vi "ExportSPadToTest.vi"(11 "Settings":T1={"Name of test"="", "Date"=timestamp(0 s since 1904-01-01), "Location"="", "Template"="", "Soundcard"="", "resolution"=32, "Sampling rate"=48000, "Ch1 Gain "=25.0, "Ch2 Gain"=10.0, "Sample time (s)"=0.3, "Pre-trigger (s)"=0.01, "Hammer Threshold"=10.0, "Positions"=12, "Taps/Position"=5, "Set Names"="", "Freq resolution"=10.0, "Hammer cutoff"=0.0, "Mic cutoff"=0.0, "Double bounce "=0.0, "Hammer Cal"=10.0, "dB Offset"=0.0, "Accel Cal"=10.0, "Vibrometer Cal"=0.0, "Mic Cal"=0.0, "Output"=2, "Voltage Cal"=1.0, "Vibrometer Port"="ASRL27::INSTR", "Range"=4, "High Pass"=2, "Bandwidth"=4, "X Range"=[], "Y Range"=[], "dB Spread"=0.0, "Trigger"=0, "Ch_1"=25, "Ch_2"=25, "flip?"=FALSE, "60Hz"=FALSE, "Time offset"=0.0, "Piezo Cal"=1.0, "Default Notes"=""} {"Ch_2" min=1 step=1; "Ch_1" min=1 max=100 step=1; "Trigger" items=["Hammer (force)", "Self-tap", "Spacebar"]; "Bandwidth" items=["1 kHz"=1, "5 kHz"=5, "10 kHz"=10, "25 kHz"=25, "50 kHz"=50, "100 kHz"=100]; "High Pass" items=["Off", "13 Hz", "104 Hz"]; "Range" items=["10 mm/s"=1, "20 mm/s"=2, "50 mm/s"=5, "100 mm/s"=10, "200 mm/s"=20, "500 mm/s"=50, "1 m/s"=100, "2 m/s"=200]; "Output" items=["Accelerometer", "Speed (from acceleration)", "Microphone", "Vibrometer", "Piezo"]; "Voltage Cal" format="%#_13g"; "Ch2 Gain" format="%#_13g"; "Ch1 Gain" format="%#_13g"; "Double bounce" min=0.0; "Mic cutoff" min=0.0 format="%#_4g"; "Hammer cutoff" min=0.0 format="%#_4g"; "Freq resolution" min=0.0; "Pre-trigger (s)" format="%#_13g"; "Date" format="%<%H:%M\n%d/%m/%y>T"; "resolution" items=["16 bit"=16, "24 bit"=24, "32 bit"=32]; "Sampling rate" items=["22050 samp/s"=22050, "44100 samp/s"=44100, "48000 samp/s"=48000]}) -> (2 "Success":bool, 3 "Settings Out":T1={"Name of test"="", "Date"=timestamp(0 s since 1904-01-01), "Location"="", "Template"="", "Soundcard"="", "resolution"=32, "Sampling rate"=48000, "Ch1 Gain "=25.0, "Ch2 Gain"=10.0, "Sample time (s)"=0.3, "Pre-trigger (s)"=0.01, "Hammer Threshold"=10.0, "Positions"=12, "Taps/Position"=5, "Set Names"="", "Freq resolution"=10.0, "Hammer cutoff"=0.0, "Mic cutoff"=0.0, "Double bounce "=0.0, "Hammer Cal"=1.0, "dB Offset"=0.0, "Accel Cal"=1.0, "Vibrometer Cal"=1.0, "Mic Cal"=1.0, "Output"=2, "Voltage Cal"=1.0, "Vibrometer Port"="ASRL27::INSTR", "Range"=4, "High Pass"=2, "Bandwidth"=4, "X Range"=[], "Y Range"=[], "dB Spread"=0.0, "Trigger"=0, "Ch_1"=1, "Ch_2"=2, "flip?"=FALSE, "60Hz"=FALSE, "Time offset"=0.0, "Piezo Cal"=1.0, "Default Notes"=""} {"Ch_2" min=1 step=1; "Ch_1" min=1 max=100 step=1; "Trigger" items=["Hammer (force)", "Self-tap", "Spacebar"]; "Bandwidth" items=["1 kHz"=1, "5 kHz"=5, "10 kHz"=10, "25 kHz"=25, "50 kHz"=50, "100 kHz"=100]; "High Pass" items=["Off", "13 Hz", "104 Hz"]; "Range" items=["10 mm/s"=1, "20 mm/s"=2, "50 mm/s"=5, "100 mm/s"=10, "200 mm/s"=20, "500 mm/s"=50, "1 m/s"=100, "2 m/s"=200]; "Output" items=["Accelerometer", "Speed (from acceleration)", "Microphone", "Vibrometer", "Piezo"]; "Voltage Cal" format="%#_13g"; "Ch2 Gain" format="%#_13g"; "Ch1 Gain" format="%#_13g"; "Double bounce" min=0.0; "Mic cutoff" min=0.0 format="%#_4g"; "Hammer cutoff" min=0.0 format="%#_4g"; "Freq resolution" min=0.0; "Pre-trigger (s)" format="%#_13g"; "Date" format="%<%H:%M\n%d/%m/%y>T"; "resolution" items=["16 bit"=16, "24 bit"=24, "32 bit"=32]; "Sampling rate" items=["22050 samp/s"=22050, "44100 samp/s"=44100, "48000 samp/s"=48000]})   [LabVIEW 2022 SP3]
uses:
  PreferencesControl.ctl
  <vilib>/Utility/miscctls.llb/LVSelectionTypeDef.ctl
  <vilib>/Utility/error.llb/Trim Whitespace One-Sided.vi
panel:
  in  "Instrument Notes":string
  in  "Instrument Name":string(combo)
  in  "Test Name":string
  out "File name":string
  in  "Tag List":bool
  in  "Instrument Keywords":string
  in  "OK Button":bool
  in  "Cancel Button":bool
  # "Export to New Test"
  # "Hz"
  # "dB"
  # "dB"
  # "sec"
  # "sec"
  # "mV/Pa"
  # "mV/m/s2"
  # "mV/mm/s"
  # "V/N"
  # "sec"
  # "sec"
  # "mV/N"
  # "a.u."
  # "a.u."
  # "sec"
  # "Hz"
  # "dB"
  # "dB"
  # "sec"
  # "sec"
  # "mV/Pa"
  # "mV/m/s2"
  # "mV/mm/s"
  # "V/N"
  # "sec"
  # "sec"
  # "mV/N"
  # "a.u."
  # "a.u."
  # "sec"
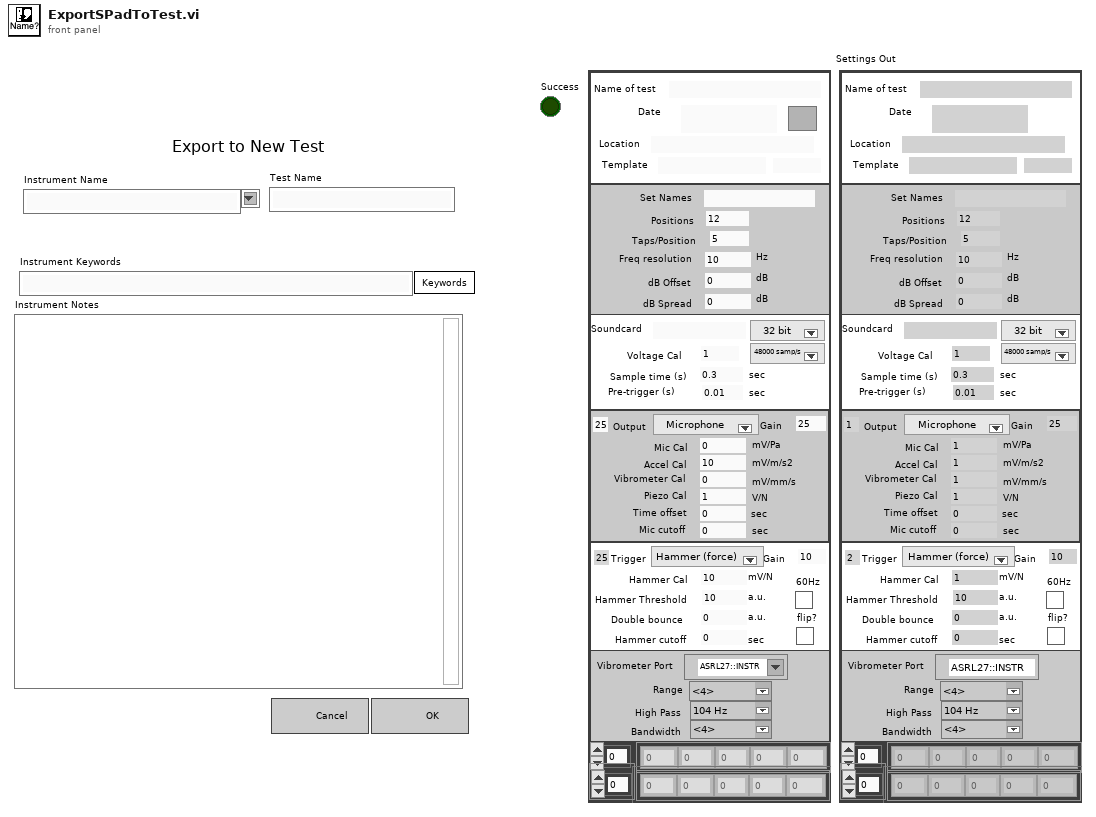
[diagram p1: front panel]
types:
  T1 = typedef "PreferencesControl.ctl" = cluster{"Name of test":string, "Date":timestamp, "Location":string, "Template":string, "Soundcard":string, "resolution":u16, "Sampling rate":u16, "Ch1 Gain ":dbl, "Ch2 Gain":dbl, "Sample time (s)":dbl, "Pre-trigger (s)":dbl, "Hammer Threshold":dbl, "Positions":i16, "Taps/Position":i16, "Set Names":string, "Freq resolution":dbl, "Hammer cutoff":dbl, "Mic cutoff":dbl, "Double bounce ":dbl, "Hammer Cal":dbl, "dB Offset":dbl, "Accel Cal":dbl, "Vibrometer Cal":dbl, "Mic Cal":dbl, "Output":u16, "Voltage Cal":dbl, "Vibrometer Port":refnum<visa-resource-name>, "Range":u16, "High Pass":u16, "Bandwidth":u16, "X Range":cluster{"Minimum":dbl, "Maximum":dbl, "Increment":dbl, "Minor Increment":dbl, "Start":dbl}[], "Y Range":cluster{"Minimum":dbl, "Maximum":dbl, "Increment":dbl, "Minor Increment":dbl, "Start":dbl}[], "dB Spread":dbl, "Trigger":u16, "Ch_1":u8, "Ch_2":u8, "flip?":bool, "60Hz":bool, "Time offset":dbl, "Piezo Cal":dbl, "Default Notes":string}
  T2 = enum8{"Enabled", "Disabled", "Disabled and Grayed Out"}
  T3 = typedef "LVSelectionTypeDef.ctl" = cluster{"Selection Start":u32, "Selection End":u32}
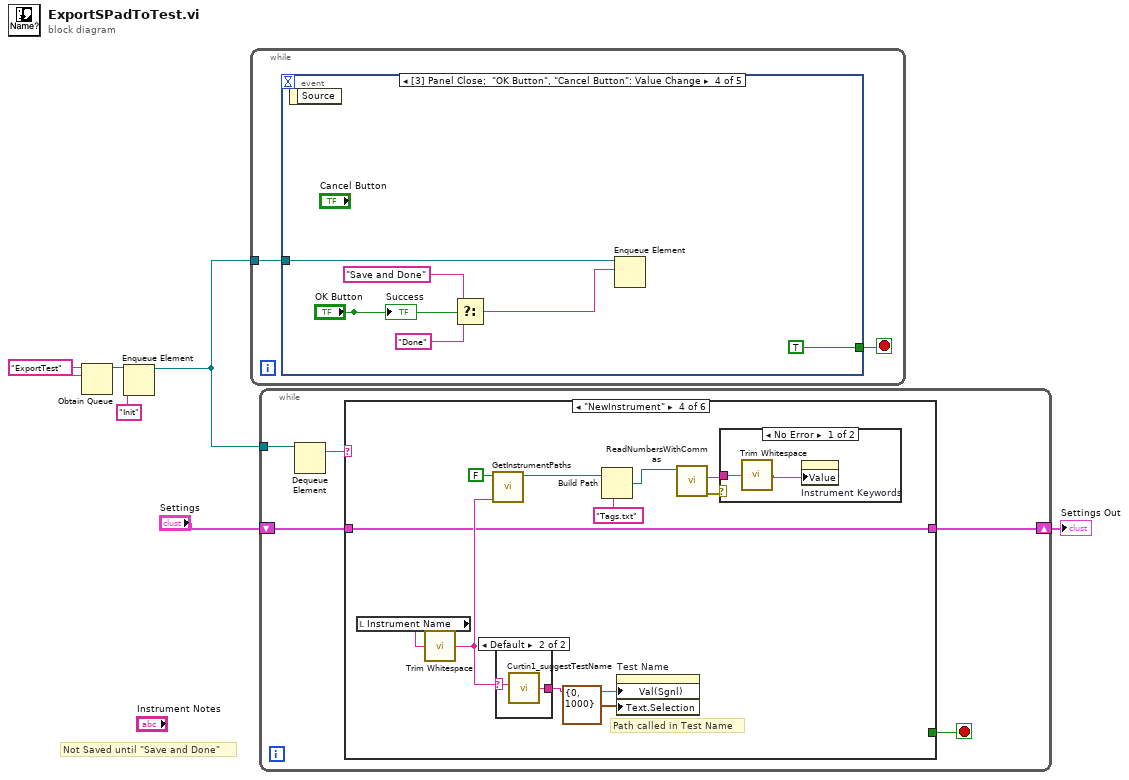
[diagram p0: block diagram]
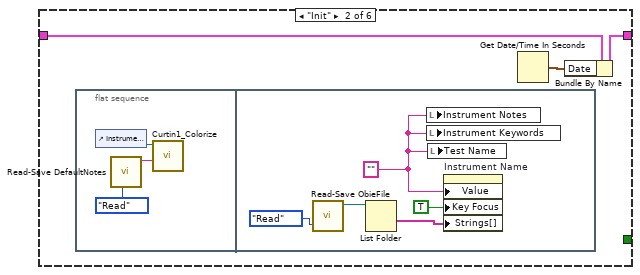
[diagram p3: hidden frame]
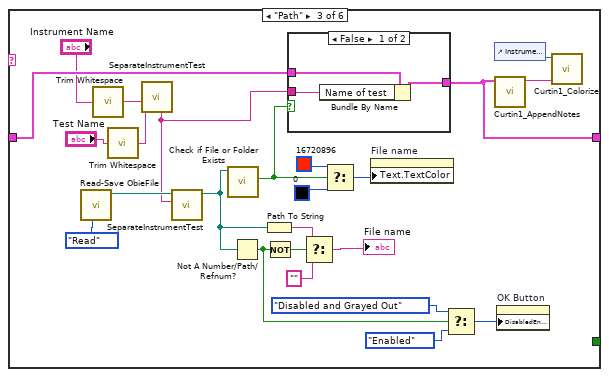
[diagram p4: hidden frame]
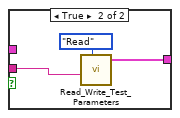
[diagram p5: hidden frame]
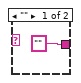
[diagram p7: hidden frame]
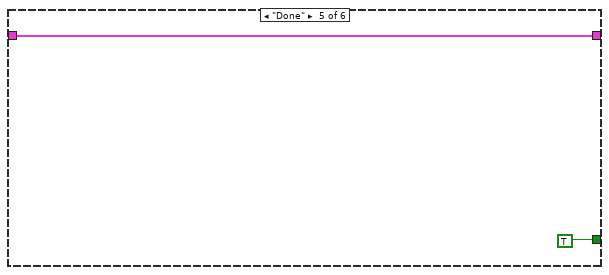
[diagram p8: hidden frame]
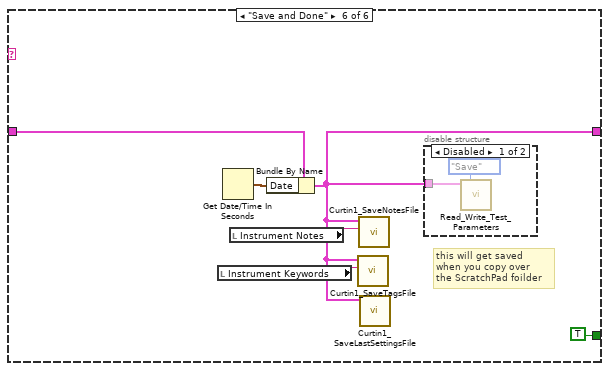
[diagram p9: hidden frame]
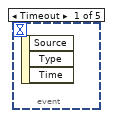
[diagram p11: hidden frame]
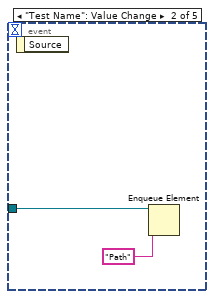
[diagram p12: hidden frame]
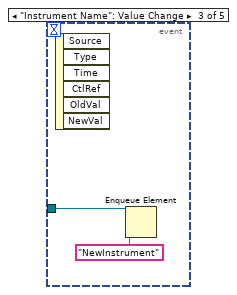
[diagram p13: hidden frame]
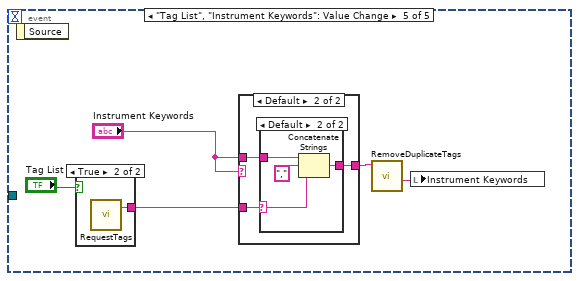
[diagram p14: hidden frame]
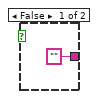
[diagram p17: hidden frame]
diagram:
  w6 = "ExportTest" ("name (unnamed)")
  # "Not Saved until \"Save and Done\""
  n1 = Obtain Queue(name (unnamed)=w6, element data type=w6) -> (queue out=w5:refnum<queue>)  [unwired: 3 in, 2 out]
  n2 = Enqueue Element(queue=w5, element="Init") -> (queue out=w3:refnum<queue>)  [unwired: 2 in, 2 out]
  n3 = while {
    tunnel: w3 -> [w7]
    stop <- w8 stop-if-true
    n4 = event shown="[3] Panel Close;  \"OK Button\", \"Cancel Button\": Value Change" {
      selector: _ -> [_ _ _ _ _]
      dyn-events: _ -> [_ _ _ _ _]
      timeout: _ -> [_ _ _ _ _]
      tunnel: [_ _ _ TRUE _] -> w8
      tunnel: w7 -> [_ w9 w11 w17 _]
      event Timeout {
        n5 = event-data() -> ()  [unwired: 1 in, 3 out]
      }
      event "Test Name": Value Change {
        n6 = event-data() -> ()  [unwired: 1 in, 1 out]
        n7 = Enqueue Element(queue=w9, element="Path") -> ()  [unwired: 2 in, 3 out]
      }
      event "Instrument Name": Value Change {
        n8 = event-data() -> ()  [unwired: 1 in, 6 out]
        n9 = Enqueue Element(queue=w11, element="NewInstrument") -> ()  [unwired: 2 in, 3 out]
      }
      event Panel Close; "OK Button", "Cancel Button": Value Change {
        n10 = event-data() -> ()  [unwired: 1 in, 1 out]
        n11 = Select(t="Save and Done" ("element"), s="OK Button", f="Done" ("element")) -> (s? t:f=w14:string)
        n12 = Enqueue Element(queue=w17, element=w14) -> ()  [unwired: 2 in, 3 out]
        "Success" <- "OK Button"
      }
      event "Tag List", "Instrument Keywords": Value Change {
        n13 = event-data() -> ()  [unwired: 1 in, 1 out]
        n14 = case shown="True" "Tag List" {
          tunnel: ["" ("Tags out") w34] -> w23
          frame False {
          }
          frame True {
            n15 = call "RequestTags.vi"() -> ("Tags out"=w34:string)  [unwired: 11 in]
          }
        }
        n16 = case shown="Default" "Instrument Keywords" {
          tunnel: w23 -> [w24 w25]
          tunnel: "Instrument Keywords" -> [_ w27]
          tunnel: [w24 w26] -> w21
          frame "" {
          }
          frame Default {
            n17 = case shown="Default" w25 {
              selector: w25 -> [_ w29]
              tunnel: w27 -> [w28 w32]
              tunnel: [w28 w31] -> w26
              frame "" {
              }
              frame Default {
                n18 = Concatenate Strings(w32, "," ("string"), w29) -> (w31:string)
              }
            }
          }
        }
        n19 = call "RemoveDuplicateTags.vi"("Tags"=w21) -> ("Tag string"=w19:string)  [unwired: 9 in, 1 out]
        n20 = local write "Instrument Keywords"(w19) -> ()
      }
    }
  }
  n21 = while {
    tunnel: w3 -> [w38]
    shift-right: [w35] -> w1
    shift-left: "Settings" -> [w36]
    stop <- w37 stop-if-true
    n22 = Dequeue Element(queue=w38) -> (element=w39:string)  [unwired: 2 in, 3 out]
    n23 = case shown="\"NewInstrument\"" w39 {
      tunnel: [_ _ _ _ TRUE TRUE] -> w37
      tunnel: w36 -> [w40 w41 w59 w85 w98 w101]
      tunnel: [w40 w43 w56 w85 w98 w100] -> w35
      frame Default {
      }
      frame "Init" {
        n24 = flat-sequence {
          frame #0 {
            n25 = control-ref of="Instrument Notes"() -> (w45:refnum<vi>)
            n26 = call "Read-Save DefaultNotes.vi"("Task"=enum16{"Save", "Read"}."Read") -> ("Notes Out"=w44:string)  [unwired: 9 in, 1 out]
            n27 = call "Curtin1_Colorize.vi"("Instrument Notes"=w44, "Text"=w45) -> ()  [unwired: 10 in]
          }
          frame #1 {
            w47 = "" ("Value (Signaling)")
            n28 = call "Read-Save ObieFile.vi"("Task"=enum16{"Save", "Read"}."Read") -> ("DataPath Out"=w50:path)  [unwired: 8 in, 2 out]
            n29 = List Folder(path=w50) -> (folder names=w51:string[])  [unwired: 3 in, 3 out]
            n30 = local write "Instrument Notes"(w47) -> ()
            n31 = local write "Instrument Keywords"(w47) -> ()
            n32 = local write "Test Name"(w47) -> ()
            n33 = property on="Instrument Name" class="CmbBox"("Value"=w47, "Key Focus"=TRUE, "Strings[]"=w51) -> ()  [unwired: 2 in, 2 out]
          }
        }
        n34 = Get Date/Time In Seconds() -> (seconds since 1Jan1904=w42:timestamp)
        n35 = Bundle By Name(cluster=w41, "Date"=w42) -> (w43:T1)
      }
      frame "Path" {
        n36 = call "Read-Save ObieFile.vi"("Task"=enum16{"Save", "Read"}."Read") -> ("DataPath Out"=w62:path)  [unwired: 8 in, 2 out]
        n37 = call <vilib>:"Trim Whitespace.vi"("string"="Instrument Name") -> ("trimmed string"=w55:string)  [unwired: 1 in]
        n38 = call <vilib>:"Trim Whitespace.vi"("string"="Test Name") -> ("trimmed string"=w52:string)  [unwired: 1 in]
        n39 = call "SeparateInstrumentTest.vi"("test in"=w52, "Instrument in"=w55) -> ("Instrument -- test out"=w60:string)  [unwired: 5 in, 4 out]
        n40 = call "SeparateInstrumentTest.vi"("Instrument"=w60, "path in"=w62) -> ("path out"=w61:path)  [unwired: 5 in, 4 out]
        n41 = call <vilib>:"Check if File or Folder Exists.vi"("path"=w61) -> ("file or folder exists?"=w64:bool)  [unwired: 8 in, 2 out]
        n42 = Not A Number/Path/Refnum?(number/path/refnum=w61) -> (NaN/Path/Refnum?=w74:bool)
        n43 = Path To String(path=w61) -> (string=w73:string)
        n44 = Not(x=w74) -> (.not. x?=w72:bool)
        n45 = case shown="False" w64 {
          tunnel: w59 -> [w78 _]
          tunnel: [w77 w79] -> w56
          tunnel: w60 -> [w76 w80]
          frame False {
            n46 = Bundle By Name(cluster=w78, "Name of test"=w76) -> (w77:T1)
          }
          frame True {
            n47 = call "Read_Write_Test_Parameters.vi"("Task"=enum16{"Save", "Read", "Clear"}."Read", "Instrument Name"=w80) -> ("Settings"=w79:T1)  [unwired: 8 in, 1 out]
          }
        }
        n48 = Select(t=w73, s=w72, f="") -> (s? t:f=→"File name":string)
        n49 = Select(t=u32 16720896, s=w64, f=u32 0) -> (s? t:f=w71:u32)
        n50 = property on="File name" class="Str"("Text.TextColor"=w71) -> ()  [unwired: 2 in, 2 out]
        n51 = Select(t=T2."Disabled and Grayed Out" ("Disabled"), s=w74, f=T2."Enabled" ("Disabled")) -> (s? t:f=w75:T2)
        n52 = control-ref of="Instrument Notes"() -> (w58:refnum<vi>)
        n53 = call "Curtin1_AppendNotes.vi"("Settings"=w56) -> ("Instrument Notes"=w57:string)  [unwired: 10 in]
        n54 = property on="OK Button" class="Bool"("DisabledEnum"=w75) -> ()  [unwired: 2 in, 2 out]
        n55 = call "Curtin1_Colorize.vi"("Instrument Notes"=w57, "Text"=w58) -> ()  [unwired: 10 in]
      }
      frame "NewInstrument" {
        # "Path called in Test Name"
        n56 = local read "Instrument Name"() -> (w88:string)
        n57 = call <vilib>:"Trim Whitespace.vi"("string"=w88) -> ("trimmed string"=w86:string)  [unwired: 1 in]
        n58 = call "GetInstrumentPaths.vi"("Instrument"=w86, "Build?"=FALSE) -> ("Path To Instrument Folder"=w87:path)  [unwired: 5 in, 4 out]
        n59 = case shown="Default" w86 {
          selector: w86 -> [_ w97]
          tunnel: ["" w96] -> w92
          frame "" {
          }
          frame Default {
            n60 = call "Curtin1_suggestTestName.vi"("instrument"=w97) -> ("Suggested Test"=w96:string)  [unwired: 10 in]
          }
        }
        n61 = Build Path(base path=w87, name or relative path="Tags.txt") -> (appended path=w82:path)
        n62 = property on="Test Name" class="Str"("Val(Sgnl)"=w92, "Text.Selection"=T3 {"Selection Start"=0, "Selection End"=1000}) -> ()  [unwired: 2 in, 2 out]
        n63 = call "ReadNumbersWithCommas.vi"("file (use dialog)"=w82) -> ("error out"=w84:errorcluster, "text"=w83:string)  [unwired: 7 in, 2 out]
        n64 = case shown="No Error" w84 {
          tunnel: w83 -> [w94 _]
          frame No Error {
            n65 = call <vilib>:"Trim Whitespace.vi"("string"=w94) -> ("trimmed string"=w93:string)  [unwired: 1 in]
            n66 = property on="Instrument Keywords" class="Str"("Value"=w93) -> ()  [unwired: 2 in, 2 out]
          }
          frame Error {
          }
        }
      }
      frame "Done" {
      }
      frame "Save and Done" {
        # "this will get saved\nwhen you copy over\nthe ScratchPad foilder"
        n67 = local read "Instrument Keywords"() -> (w102:string)
        n68 = Get Date/Time In Seconds() -> (seconds since 1Jan1904=w104:timestamp)
        n69 = local read "Instrument Notes"() -> (w103:string)
        n70 = Bundle By Name(cluster=w101, "Date"=w104) -> (w100:T1)
        n71 = call "Curtin1_SaveTagsFile.vi"("Tags"=w102, "Settings in"=w100) -> ()  [unwired: 10 in]
        n72 = call "Curtin1_SaveNotesFile.vi"("Notes"=w103, "Settings in"=w100) -> ()  [unwired: 10 in]
        n73 = call "Curtin1_SaveLastSettingsFile.vi"("Settings in"=w100) -> ()  [unwired: 11 in]
        n74 = disable-structure shown="Disabled" {
          disable-tunnel: w100 -> [w106 _]
          frame Disabled {
            n75 = call "Read_Write_Test_Parameters.vi"("Task"=enum16{"Save", "Read", "Clear"}."Save", "Settings"=w106) -> ()  [unwired: 8 in, 2 out]
          }
          frame Enabled {
          }
        }
      }
    }
  }
  "Settings Out" <- w1
